vi "workingPicture.vi"(4 "Title":string, 5 "Image Type":u32(ring) items=["8 bits", "16 bits", "Float", "Complex", "RGB", "HSL"], 6 "File Path":path, 7 "Palette Number (gray)":T2(ring), 8 "error out 2":errorcluster, 9 "Image In":T1, 10 "Enum 2":T3(ring)) -> (0 "error out":errorcluster, 1 "Title 2":string, 2 "Image Out":T1)   [LabVIEW 2009]
uses:
  <vilib>/vision/Image Controls.llb/IMAQ Image.ctl
  <vilib>/vision/NI_Vision_Development_Module.lvlib
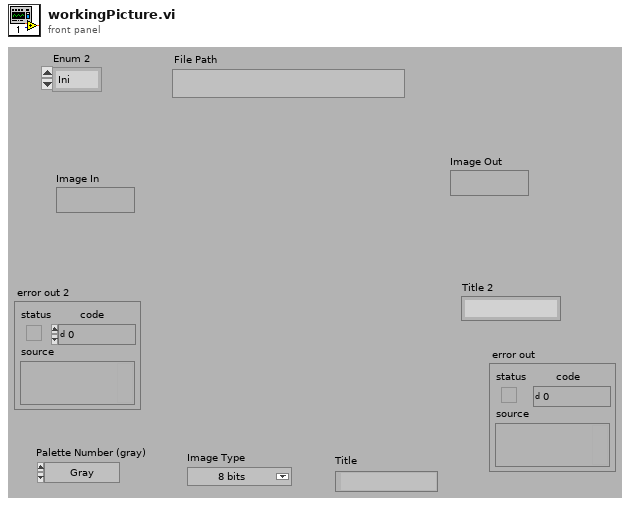
[diagram p1: front panel]
types:
  T1 = typedef "IMAQ Image.ctl" = refnum<image>
  T2 = enum32{"Gray", "Binary", "Gradient", "Rainbow", "Temperature"}
  T3 = enum16{"Ini", "Load", "Save as", "Get", "draw", "set", "dump", "convert", "colorpal", "get", "newname"}
  T4 = enum16{"Ini", "Load", "Save as", "Get", "draw", "set"}
  T5 = enum16{"Ini", "Load", "Save as", "Get", "draw", "set", "dump", "convert", "colorpal", "get"}
  T6 = enum16{"Ini", "Load", "Save as", "Get", "draw", "set", "dump", "convert", "colorpal"}
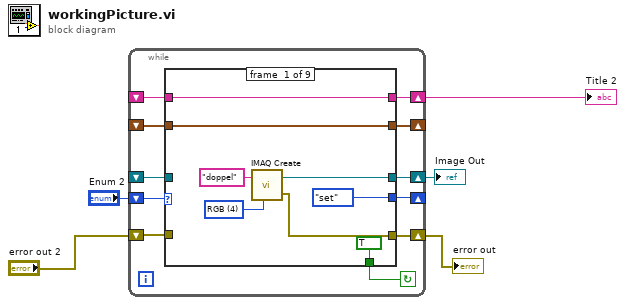
[diagram p0: block diagram]
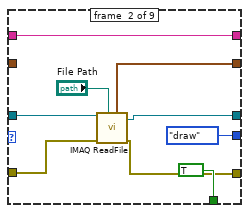
[diagram p2: hidden frame]
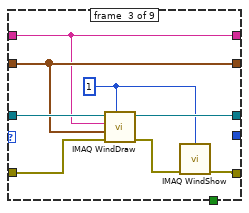
[diagram p3: hidden frame]
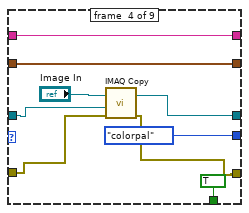
[diagram p4: hidden frame]
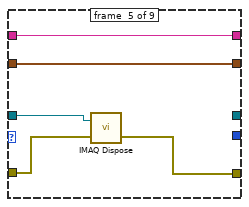
[diagram p5: hidden frame]
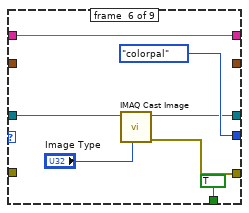
[diagram p6: hidden frame]
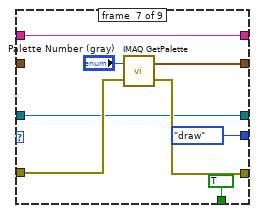
[diagram p7: hidden frame]
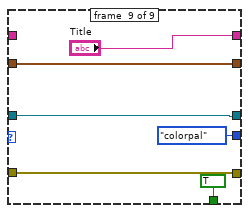
[diagram p9: hidden frame]
diagram:
  n1 = while {
    shift-right: [w16] -> w3
    shift-left: _ -> [w15]
    shift-right: [w13] -> _
    shift-left: "Enum 2" -> [w14]
    shift-right: [w11] -> _
    shift-left: _ -> [w10]
    shift-right: [w9] -> w4
    shift-left: "error out 2" -> [w8]
    shift-right: [w7] -> w2
    shift-left: _ -> [w6]
    stop <- w12 continue-if-true
    n2 = case shown="\"set\"" w14 {
      tunnel: [w24 w29 w40 w42 _ w60 w63 w72 w78] -> w16
      tunnel: w15 -> [_ w33 w41 w45 w54 w57 w63 w72 w78]
      tunnel: [T4."set" ("Enum 2") enum16{"Ini", "Load", "Save as", "Get", "draw"}."draw" ("Enum") _ T5."colorpal" ("Enum 2") _ T6."colorpal" ("Enum 2") T3."draw" ("Enum 2") _ T5."colorpal" ("Enum 2")] -> w13
      tunnel: [TRUE TRUE _ TRUE _ TRUE TRUE _ TRUE] -> w12
      tunnel: [w19 w30 w39 w48 w51 _ w69 w73 w79] -> w11
      tunnel: w10 -> [w19 _ w39 w48 w51 _ _ w73 w79]
      tunnel: [w18 w27 w36 w43 w53 w56 w68 w71 w77] -> w9
      tunnel: w8 -> [_ w26 w38 w44 w55 _ w67 w71 w77]
      tunnel: [w17 w25 w37 w49 w52 w58 w66 w74 "Title"] -> w7
      tunnel: w6 -> [w17 w25 w37 w49 w52 w58 w66 w74 _]
      frame #0 {
        w22 = u32 4 items=["8 bits", "16 bits", "Float", "Complex", "RGB", "HSL"] ("Image Type")
        n3 = call "IMAQ Create"("Image Name"="doppel", "Image Type"=w22) -> ("New Image"=w24:T1, "error out"=w18:errorcluster)  [unwired: 3 in]
      }
      frame #1 {
        n4 = call "IMAQ ReadFile"("File Path"="File Path", "error in (no error)"=w26, "Image"=w33) -> ("error out"=w27:errorcluster, "Image Out"=w29:T1, "Color Palette out"=w30:cluster{"Red":u8, "Green":u8, "Blue":u8}[])  [unwired: 4 in, 2 out]
      }
      frame #2 {
        w34 = 1 ("Window Number (0...15)")
        n5 = call "IMAQ WindDraw"("Window Number (0...15)"=w34, "error in (no error)"=w38, "Color Palette"=w39, "Title"=w37, "Image"=w41) -> ("error out"=w35:errorcluster, "Image Out (duplicate)"=w40:T1)  [unwired: 5 in]
        n6 = call "IMAQ WindShow"("error in (no error)"=w35, "Window Number (0...15)"=w34) -> ("error out"=w36:errorcluster)  [unwired: 4 in, 2 out]
      }
      frame #3 {
        n7 = call "IMAQ Copy"("error in (no error)"=w44, "Image Dst"=w45, "Image Src"="Image In") -> ("error out"=w43:errorcluster, "Image Dst Out"=w42:T1)  [unwired: 3 in]
      }
      frame #4 {
        n8 = call "IMAQ Dispose"("Image"=w54, "error in (no error)"=w55) -> ("error out"=w53:errorcluster)  [unwired: 4 in]
      }
      frame #5 {
        n9 = call "IMAQ Cast Image"("Image Type"="Image Type", "Image Src"=w57) -> ("error out"=w56:errorcluster, "Image Dst Out"=w60:T1)  [unwired: 8 in]
      }
      frame #6 {
        n10 = call "IMAQ GetPalette"("Palette Number (gray)"="Palette Number (gray)", "error in (no error)"=w67) -> ("Color Palette"=w69:cluster{"Red":u8, "Green":u8, "Blue":u8}[], "error out"=w68:errorcluster)  [unwired: 3 in]
      }
      frame #7 {
      }
      frame #8 {
      }
    }
  }
  "Image Out" <- w3
  "Title 2" <- w2
  "error out" <- w4
